vi "Register.vi"(8 "error in":errorcluster, 10 "TPCANHandle":T1 items=["PCAN_NONEBUS"=0, "PCAN_USBBUS1"=81, "PCAN_USBBUS2"=82, "PCAN_USBBUS3"=83, "PCAN_USBBUS4"=84, "PCAN_USBBUS5"=85, "PCAN_USBBUS6"=86, "PCAN_USBBUS7"=87, "PCAN_USBBUS8"=88, "PCAN_USBBUS9"=1289, "PCAN_USBBUS10"=1290, "PCAN_USBBUS11"=1291, "PCAN_USBBUS12"=1292, "PCAN_USBBUS13"=1293, "PCAN_USBBUS14"=1294, "PCAN_USBBUS15"=1295, "PCAN_USBBUS16"=1296], 11 "Read Event in":refnum<class "Read Event.lvclass">) -> (0 "error out":errorcluster, 3 "Read Event out":refnum<class "Read Event.lvclass">)   [LabVIEW 2018, in "PCANBasic.lvlib" / "Read Event.lvclass"]
uses:
  Read Event.lvclass
  Read Event.lvclass/Read Event.ctl
  Win32 Event/Win32 Event.lvclass
  Message Waiter/Message Waiter.lvclass
  epoll/epoll.lvclass
  TPCANHandle.ctl
  PCANBasic.lvlib
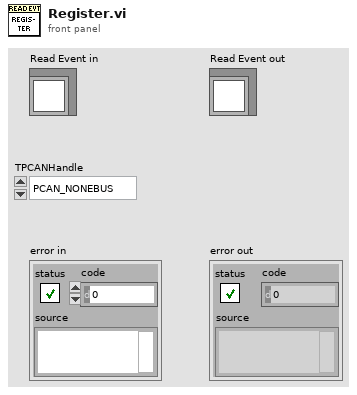
[diagram p1: front panel]
types:
  T1 = typedef "PCANBasic.lvlib/TPCANHandle.ctl" = u16
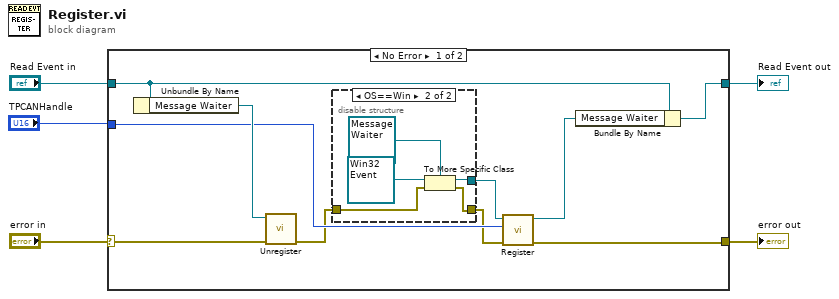
[diagram p0: block diagram]
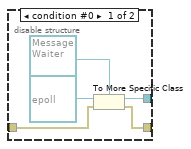
[diagram p2: hidden frame]
diagram:
  n1 = case shown="No Error" "error in" {
    selector: "error in" -> [w14 w27]
    tunnel: [w12 w27] -> w5
    tunnel: "Read Event in" -> [w11 w26]
    tunnel: [w10 w26] -> w2
    tunnel: "TPCANHandle" -> [w9 _]
    frame No Error {
      n2 = Unbundle By Name(w11) -> ("Message Waiter"=w15:refnum<class "Message Waiter.lvclass">)
      n3 = call-dynamic "Unregister.vi"("error in"=w14, "Message Waiter in"=w15) -> ("error out"=w7:errorcluster)  [unwired: 8 in, 1 out]
      n4 = disable-structure shown="OS==Win" {
        disable-tunnel: [w18 w24] -> w13
        disable-tunnel: w7 -> [w17 w22]
        disable-tunnel: [w16 w21] -> w6
        frame condition #0 {
          n5 = To More Specific Class(target class=refnum<class "Message Waiter.lvclass"> refnum ("PCANBasic.lvlib:IWait for Message.lvclass"), reference=refnum<class "epoll.lvclass"> refnum ("PCANBasic.lvlib:epoll.lvclass"), error in=w17) -> (specific class reference=w18:refnum<class "Message Waiter.lvclass">, error out=w16:errorcluster)
        }
        frame condition #1 (active) {
          n6 = To More Specific Class(target class=refnum<class "Message Waiter.lvclass"> refnum ("PCANBasic.lvlib:IWait for Message.lvclass"), reference=refnum<class "Win32 Event.lvclass"> refnum ("PCANBasic.lvlib:Win32 Event.lvclass"), error in=w22) -> (specific class reference=w24:refnum<class "Message Waiter.lvclass">, error out=w21:errorcluster)
        }
      }
      n7 = call-dynamic "Register.vi"("error in"=w6, "TPCANHandle"=w9, "Message Waiter in"=w13) -> ("error out"=w12:errorcluster, "Message Waiter out"=w8:refnum<class "Message Waiter.lvclass">)  [unwired: 7 in]
      n8 = Bundle By Name(cluster=w11, "Message Waiter"=w8) -> (w10:refnum<class "Read Event.lvclass">)
    }
    frame Error {
    }
  }
  "error out" <- w5
  "Read Event out" <- w2
